vi "Create Becker-Hickl Parameters Enum.vi"() -> ()   [LabVIEW 2021, in "Becker-Hickl Files.lvlib"]
uses:
  Becker-Hickl Files.lvlib
  Utilities/ArrayToEnum/ControlTypes__A2E.ctl
  Utilities/Utilities.lvlib
  <userlib>/_OpenG.lib/string/string.llb/openg_string.lvlib
panel:
  in  "B&H String":string="  SYS_PARA_BEGIN:\n  #PR [PR_PDEV,I,2]\n  #PR [PR_PPORT,I,2]\n  #PR [PR_PWHAT,I,1]\n  #PR [PR_PF,B,0]\n  #PR [PR_PFNAME,S,D:\\SPC400\\APPLICAT\\LW_CVI\\IMAGE.PRT]\n  #PR [PR_PORIEN,I,1]\n  #PR [PR_PEJECT,B,1]\n  #PR [PR_PWIDTH,F,100]\n  #PR [PR_PHEIGH,F,100]\n  #PR [PR_PFULL,B,1]\n  #PR [PR_PAUTO,B,1]\n  #PR [PR_STP_FN,S,C:\\PROGRAM FILES\\BH\\SPCM\\STP.CFG]\n  #PR [PR_SAVE_T,I,0]\n  #PR [PR_SLEEP,I,5]\n  #SP [SP_MODE,I,10]\n  #SP [SP_CFD_LL,F,-100]\n  #SP [SP_CFD_LH,F,5.019608]\n  #SP [SP_CFD_ZC,F,0]\n  #SP [SP_CFD_HF,F,5]\n  #SP [SP_SYN_ZC,F,0]\n  #SP [SP_SYN_FD,I,2]\n  #SP [SP_SYN_FQ,F,-200]\n  #SP [SP_SYN_HF,F,4]\n  #SP [SP_TAC_R,F,6.0122041e-08]\n  #SP [SP_TAC_G,I,1]\n  #SP [SP_TAC_OF,F,0]\n  #SP [SP_TAC_LL,F,18.82353]\n  #SP [SP_TAC_LH,F,90.588234]\n  #SP [SP_TAC_TC,F,1.4678233e-11]\n  #SP [SP_TAC_TD,F,6.0122041e-09]\n  #SP [SP_ADC_RE,I,4096]\n  #SP [SP_EAL_DE,I,0]\n  #SP [SP_NCX,I,8]\n  #SP [SP_NCY,I,1]\n  #SP [SP_PAGE,I,1]\n  #SP [SP_COL_T,F,1000]\n  #SP [SP_REP_T,F,1000]\n  #SP [SP_DIS_T,F,0.1]\n  #SP [SP_REPEAT,B,1]\n  #SP [SP_STOPT,B,1]\n  #SP [SP_OVERFL,C,N]\n  #SP [SP_WL_STA,F,500]\n  #SP [SP_WL_STO,F,551.09998]\n  #SP [SP_WL_STE,F,0.1]\n  #SP [SP_EXTST,B,0]\n  #SP [SP_STEPS,I,1]\n  #SP [SP_OFFSET,F,0]\n  #SP [SP_YWIN_N,I,8]\n  #SP [SP_XWIN_N,I,8]\n  #SP [SP_TWIN_N,I,1]\n  #SP [SP_X_EQU,B,1]\n  #SP [SP_Y_EQU,B,1]\n  #SP [SP_T_EQU,B,1]\n  #SP [SP_DITH,I,128]\n  #SP [SP_EN_INT,B,0]\n  #SP [SP_INCR,I,1]\n  #SP [SP_DAES,B,0]\n  #SP [SP_SPE_FN,S,d:\\eitan\\03_24_2014\\dsdna_d7_1.spc]\n  #SP [SP_CYCLES,U,1]\n  #SP [SP_DAEC,B,0]\n  #SP [SP_MEM_BANK,I,0]\n  #SP [SP_DTCOMP,B,1]\n  #SP [SP_SCF,I,0]\n  #SP [SP_POL_L,I,1]\n  #SP [SP_POL_F,I,1]\n  #SP [SP_PIX,I,0]\n  #SP [SP_LDIV,I,2]\n  #SP [SP_ACCUM,B,0]\n  #SP [SP_ROUT,B,0]\n  #SP [SP_TAC_EH,F,10]\n  #SP [SP_DLIM,I,204800]\n  #SP [SP_PHOT_F,U,34952533]\n  #SP [SP_EN_DLIM,B,1]\n  #SP [SP_PH_BUF,I,204800]\n  #SP [SP_FLB_Y,I,0]\n  #SP [SP_FLB_X,I,0]\n  #SP [SP_BORD_U,I,1]\n  #SP [SP_BORD_L,I,6]\n  #SP [SP_POL_P,I,1]\n  #SP [SP_PIX_T,F,2e-07]\n  #SP [SP_PIX_CLK,I,1]\n  #SP [SP_TRIGGER,I,16]\n  #SP [SP_SCAN_X,I,32]\n  #SP [SP_SCAN_Y,I,32]\n  #SP [SP_SCAN_RX,I,1]\n  #SP [SP_SCAN_RY,I,1]\n  #SP [SP_FIF_TYP,I,1]\n  #SP [SP_EPX_DIV,I,4]\n  #SP [SP_MTCLK,I,0]\n  #SP [SP_ADD_SEL,I,0]\n  #SP [SP_SXWIN_N,I,8]\n  #SP [SP_SYWIN_N,I,8]\n  #SP [SP_SX_EQU,B,1]\n  #SP [SP_SY_EQU,B,1]\n  #SP [SP_ASAVE,I,32]\n  #SP [SP_ADC_ZOOM,I,0]\n  #SP [SP_FIF_FNO,I,1]\n  #SP [SP_FCYCLES,U,1]\n  #SP [SP_XY_GAIN,I,1]\n  #SP [SP_IMG_X,I,128]\n  #SP [SP_IMG_Y,I,128]\n  #SP [SP_IMG_RX,I,1]\n  #SP [SP_IMG_RY,I,1]\n  #SP [SP_MST_CLK,I,0]\n  #SP [SP_ADC_DE,I,0]\n  #SP [SP_DET_TYP,I,0]\n  #SP [SP_X_AXIS,I,0]\n  #SP [SP_CH_EN,I,4191231]\n  #SP [SP_CH_SL,I,16777215]\n  #SP [SP_CH_F1,I,0]\n  #SP [SP_CH_F2,I,136314880]\n  #DI [DI_SCALE,I,1]\n  #DI [DI_MAXCNT,L,65000]\n  #DI [DI_LBLINE,L,1]\n  #DI [DI_BLINE,L,0]\n  #DI [DI_GRID,B,1]\n  #DI [DI_GCOL_F,I,14737632]\n  #DI [DI_GCOL_B,I,16777215]\n  #DI [DI_TRACE,I,0]\n  #DI [DI_BOD_C,I,32896]\n  #DI [DI_2DDIS,I,0]\n  #DI [DI_2DTRNO,I,3]\n  #DI [DI_3DOFFX,I,3]\n  #DI [DI_3DOFFY,I,1]\n  #DI [DI_3DINCX,I,0]\n  #DI [DI_3DCOL,I,0]\n  #DI [DI_3DMODE,I,3]\n  #DI [DI_YWIN,I,1]\n  #DI [DI_XWIN,I,1]\n  #DI [DI_TWIN,I,1]\n  #DI [DI_PSTYLE,I,1]\n  #DI [DI_PFREQ,I,1]\n  #DI [DI_CUR,B,0]\n  #DI [DI_RATE,B,1]\n  #DI [DI_2DC1,B,1]\n  #DI [DI_2DC2,B,1]\n  #DI [DI_2DC1C,I,10]\n  #DI [DI_2DC2C,I,13]\n  #DI [DI_2DC1S,I,0]\n  #DI [DI_2DC2S,I,0]\n  #DI [DI_3DC1C,I,12]\n  #DI [DI_3DC2C,I,14]\n  #DI [DI_SIZE,I,0]\n  #DI [DI_3DSTYL,I,1]\n  #DI [DI_INTCOL,I,1]\n  #DI [DI_INTPIX,I,1]\n  #DI [DI_COL_NO,I,3]\n  #DI [DI_COLMIN,I,0]\n  #DI [DI_COLMAX,I,16777215]\n  #DI [DI_COL2,I,65280]\n  #DI [DI_COL3,I,255]\n  #DI [DI_COL4,I,13408716]\n  #DI [DI_COL5,I,13421823]\n  #DI [DI_HICOL,I,16711680]\n  #DI [DI_XREV,B,0]\n  #DI [DI_YREV,B,0]\n  #DI [DI_DETAIL,B,1]\n  #DI [DI_SYWIN,I,3]\n  #DI [DI_SXWIN,I,1]\n  #DI [DI_ASCALE,I,1]\n  SYS_PARA_END:\n  TRACE_PARA_BEGIN:\n  #TR #0 [1,3342591,1,1,4,1,1,1]\n  #TR #1 [1,52224,5,1,1,2,1,5]\n  #TR #2 [1,16711680,7,1,1,3,1,7]\n  #TR #3 [0,13382655,1,1,1,4,1,1]\n  #TR #4 [0,16711935,1,1,1,1,1,1]\n  #TR #5 [0,3342591,1,1,1,1,1,1]\n  #TR #6 [0,0,1,1,1,1,1,1]\n  #TR #7 [0,8388608,3,1,1,1,1,1]\n  TRACE_PARA_END:\n  WIND_PARA_BEGIN:\n  #WI #0 *NO *0 [0,31]\n  #WI #0 *NO *1 [32,63]\n  #WI #0 *NO *2 [64,95]\n  #WI #0 *NO *3 [96,127]\n  #WI #0 *NO *4 [128,159]\n  #WI #0 *NO *5 [160,191]\n  #WI #0 *NO *6 [192,223]\n  #WI #0 *NO *7 [224,255]\n  #WI #1 *NO *0 [0,0]\n  #WI #1 *NO *1 [0,0]\n  #WI #1 *NO *2 [0,0]\n  #WI #1 *NO *3 [0,0]\n  #WI #1 *NO *4 [0,0]\n  #WI #1 *NO *5 [0,0]\n  #WI #1 *NO *6 [0,0]\n  #WI #1 *NO *7 [0,0]\n  #WI #2 *NO *0 [0,4095]\n  WIND_PARA_END:"
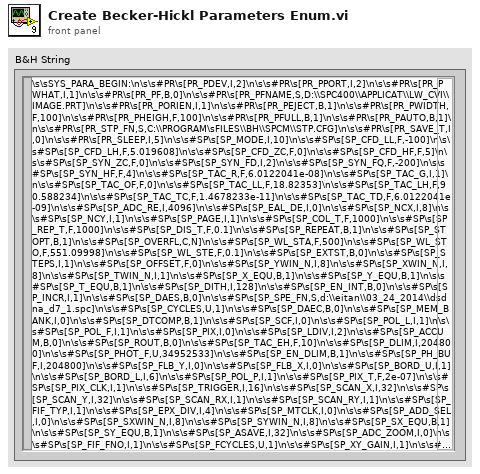
[diagram p1: front panel]
types:
  T1 = typedef "Utilities.lvlib/ControlTypes__A2E.ctl" = enum32{"not a control VI", "control", "typedef", "strict typedef"}
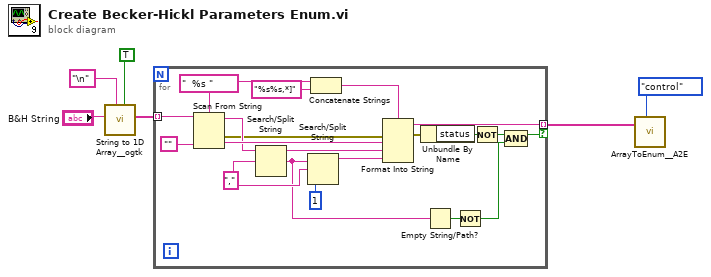
[diagram p0: block diagram]
diagram:
  n1 = call <userlib>:"String to 1D Array__ogtk.vi"("ignore duplicate delimiters? (F=No)"=TRUE, "delimiter (Tab)"="\n", "string"="B&H String") -> ("Array of Strings"=w4:string[])  [unwired: 8 in]
  n2 = for {
    tunnel: w4 -> [w20] mode=indexing
    tunnel: [w24] -> w2 mode=indexing if=w10
    w13 = "," ("search string/char (-)")
    w17 = "  %s " ("format string")
    n3 = Scan From String(format string=w17, input string=w20, default 1="") -> (remaining string=w16:string, error out=w11:errorcluster, output 1=w18:string)  [unwired: 2 in, 1 out]
    n4 = Search/Split String(string=w16, search string/char (-)=w13) -> (substring before match=w15:string, match + rest of string=w9:string)  [unwired: 1 in, 1 out]
    n5 = Search/Split String(string=w9, search string/char (-)=w13, offset (0)=1) -> (substring before match=w12:string)  [unwired: 2 out]
    n6 = Concatenate Strings(w17, "%s%s,*]" ("string")) -> (w25:string)
    n7 = Format Into String(format string=w25, error in=w11, w18, w15, w12) -> (resulting string=w24:string, error out=w23:errorcluster)  [unwired: 1 in]
    n8 = Unbundle By Name(w23) -> ("status"=w22:bool)
    n9 = Empty String/Path?(string/path=w9) -> (empty?=w8:bool)
    n10 = Not(x=w8) -> (.not. x?=w7:bool)
    n11 = Not(x=w22) -> (.not. x?=w21:bool)
    n12 = Compound Arithmetic op=AND(w21, w7) -> (w10:bool)
  }
  n13 = call "ArrayToEnum__A2E.vi"("Control VI Type (control)"=ControlTypes__A2E."control", "Enum Strings"=w2) -> ()  [unwired: 9 in, 1 out]
